vi "Float32 Destroy.vi"(8 "error in (no error)":errorcluster, 11 "Float32 DVR in":refnum<data-value>) -> (0 "error out":errorcluster)   [LabVIEW 2012, in "MDSplus.lvlib"]
uses:
  <vilib>/MDSplus/Library/MDSplus.lvlib
  <vilib>/MDSplus/Classes/Data_Class/Scalar_Class/Float32_Class/Float32.lvclass
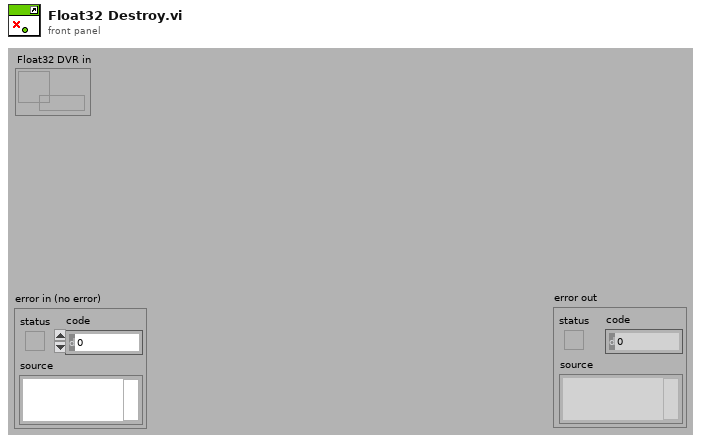
[diagram p1: front panel]
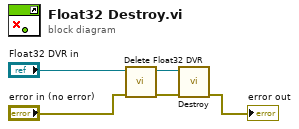
[diagram p0: block diagram]
diagram:
  n1 = call <vilib>:"Delete Float32 DVR.vi"("error in (no error)"="error in (no error)", "Float32 DVR in"="Float32 DVR in") -> ("error out"=w2:errorcluster, "Float32 out"=w3:refnum<class "Float32.lvclass">)  [unwired: 8 in]
  n2 = call-dynamic "Destroy.vi"("error in (no error)"=w2, "Float32 in"=w3) -> ("error out"=→"error out":errorcluster)  [unwired: 9 in]
